vi "Read N.vi"(9 "ForLoop in":refnum<class "WhileLoop.lvclass">) -> (3 "ForLoop out":refnum<class "WhileLoop.lvclass">, 4 "N":refnum<class "Tunnel.lvclass">)   [LabVIEW 2014]
uses:
  WhileLoop.lvclass
  Tunnel/Tunnel.lvclass
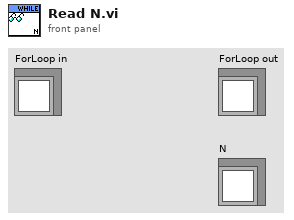
[diagram p1: front panel]
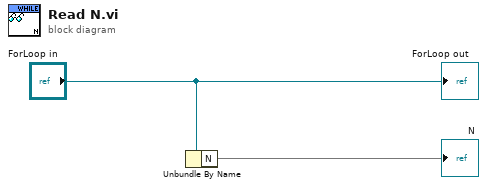
[diagram p0: block diagram]
diagram:
  n1 = Unbundle By Name("ForLoop in") -> ("N"=→"N")
  "ForLoop out" <- "ForLoop in"
